vi "VisBx Anzeige.vi"() -> ()   [LabVIEW 2020, in "Anlagenuebersicht.lvlib"]
uses:
  Seiten/Anlagenuebersicht/VisBx Anzeige/Anlagenuebersicht.lvlib
  Visualisierungs Elemente/Zahlen-Ausgabefeld.ctl
  Seiten/Anlagenuebersicht/Aktionen Ausgabefaelder einfaerben.ctl
  <vilib>/Utility/miscctls.llb/LVPointTypeDef.ctl
  Seiten/Anlagengrenzwerte/FGV Anlagengrenzwerte Aktionen.ctl
  Seiten/FT-IR/FGV FT-IR Gasliste Aktionen.ctl
  PNS/Aktionen FGV Grenzwerte.ctl
  Seiten/System Einstellungen V2/Aktioen FGV System.ctl
  Seiten/FT-IR/FGV FT-IR Diagnose Aktionen.ctl
  Messdaten/Aktionen FGV Messdaten.ctl
  Amium PNS/Aktion FGV Amium Daten.ctl
  PNS/Aktionen FGV Istwerte.ctl
  Stoerungen/Stoerungen Messgeraet/Aktionen Kommunikation Stoerung.ctl
  Funktionstasten/FGV Erweiterte Bedienung Aktion.ctl
  <vilib>/picture/picture.llb/Draw True-Color Pixmap.vi
  Seiten/Erweiterte Konfig/Konfig CG-Check/CG-Test.vi
  Seiten/Anlagenuebersicht/VisBx Anzeige/VisBx Anzeige.lvlib
  Seiten/Anlagenuebersicht/VisBx Anzeige/TDMS laden/TDMS laden.lvlib
  Allgemein/allgemeine Sub-VIs.lvlib
  cRIO/PC/Kommunikation mit cRIO.lvlib
  Seiten/FT-IR/FT-IR.lvlib
  Stoerungen/Stoerungen.lvlib
  Seiten/Anlagengrenzwerte/Anlagengrenzwerte.lvlib
  Funktionstasten/Funktionstasten.lvlib
  Messdaten/Messdaten.lvlib
  PNS/PNS.lvlib
  Seiten/System Einstellungen V2/System Einstellungen V2.lvlib
  Seiten/Erweiterte Konfig/Konfig CG-Check/CG-Check Konfig.lvlib
  Amium PNS/Amium PNS.lvlib
  Amium PNS/Anlagenuebersicht_amium2.vi
panel:
  out "16B1":string="LS\n\n-16B1" caption="-21Y8"
  out "N2Exh 2":string="N2\nEXH"
  out "-22Y3 50l 2":string="-22Y3" caption="-21Y8"
  out "17B3 50l":string="LS\n\n-17B3" caption="-21Y8"
  out "17B2 50l":string="LS\n\n-17B2" caption="-21Y8"
  out "16B2 50l":string="LS\n\n-16B2" caption="-21Y8"
  out "16B2":string="LS\n\n-16B2" caption="-21Y8"
  out "-22Y1 50l":string="-22Y1" caption="-21Y8"
  out "-22Y1":string="-22Y1" caption="-21Y8"
  out "PR0,2":string="PR\n0,3bar"
  out "PA3":string="PA\n3"
  out "N2Exh":string="N2\nEXH"
  out "-23Y8":string="-23Y8"
  out "-21Y7":string="-21Y7"
  out "-21Y8":string="-21Y8"
  out "Umgebungstemperatur:":T1 format="%.1f"
  out "Boolesch":bool
  out "HL Ext. SP1:":T1 format="%.1f"
  in  "VFS":bool
  in  "VFS - Inaktiv":bool
  in  "VFS - FEHLER":bool
  in  "VFS - Aktiv":bool=TRUE
  out "kPa":T1 caption="Messgasdruck Amium"
  out "Durchflussblock":T1 caption="Durchflussblock:" format="%.1f"
  out "Druck Filterblock:":T1
  in  "CG-Test":bool caption="Dichtheitstest"
  out "Umgebungsdruck:":T1
  out "Druck Ausgang:":T1
  out "Durchfluss Bypass:":T1 caption="Flow Bypass:" format="%.1f"
  out "HL zu FID:":T1 format="%.1f"
  out "Filterblock PNS":T1 caption="Filterblock:" format="%.1f"
  out "Heizleitung SP2:":T1 caption="HL SP2:" format="%.1f"
  out "Heizleitung SP1:":T1 caption="HL SP1:" format="%.1f"
  out "Gaskühler 2":T1 caption="Gaskühler:" format="%.1f"
  out "Gaskühler":T1 caption="Gaskühler:" format="%.1f"
  out "Flow PMA:":T1 caption="Fluss PMD:" format="%.1f"
  out "Taupunkt":T1 caption="Taupunkt:" format="%.1f"
  out "Druck Kalter Block":T1 caption="Druck Kalter Block:"
  out "O2":T1 caption="O2:" format="%.2f"
  out "H2O":T1 format="%.2f"
  out "HC":T1 caption="HC:"
  in  "N2 zu PNS":bool
  out "Heizung VFE2:":T1 format="%.1f"
  out "HL Ext. SP2:":T1 format="%.1f"
  out "Schaltschrank:":T1 format="%.1f"
  out "Druck CalGas:":T1 format="%.1f"
  out "HL zu Filter:":T1 format="%.1f"
  out "HL zu FT-IR:":T1 format="%.1f"
  out "Filter:":T1 format="%.1f"
  out "Pumpe:":T1 format="%.1f"
  out "Betriebsstunden Pumpe:":T1 format="%.1f"
  out "Betriebsstunden Anlage:":T1 caption="Betriebsstunden Anlage / FTIR:" format="%.1f"
  out "Temp. Messzelle:":T1 format="%.1f"
  out "Eingangsdruck FT-IR:":T1 format="%.3f"
  out "Durchfluss FT-IR:":T1 format="%.1f"
  out "Aktive Störungen":string[](array[string])
  in  "Fehler":string="Die Umgebungsvariable besitzt\nnicht den selben Datentyp wie\ndie TDMS-Datei."
  out "Bild":picture
  # "Anlagenübersicht"
  # "SPAN 1"
  # "-23Y1"
  # "SPAN 2"
  # "-23Y6"
  # "PS"
  # "-23Y2"
  # "SPAN 3"
  # "0-10"
  # "bar"
  # "-22Y2"
  # "-23Y3"
  # "-35B5"
  # "N2.....Stickstoff Gasförmig\nCA.....Druckluft\nCG.....Cal. Gas\nAA.....Umgebungs Luft\nPA.....Spülluft FT-IR\n\nPR....Druckregler\nPS....Druckschalter\nFS....Flow Regler\nLS....Levelsensor\nFM...Flow Sensor"
  # "-35B1"
  # "-23Y4"
  # "FM"
  # "-43Y1"
  # "S"
  # "-21Y5"
  # "FTIR"
  # "-35B2"
  # "-11Y7"
  # "-11Y3"
  # "SP1"
  # "-11Y5"
  # "-11Y6"
  # "SP2"
  # "-11Y2"
  # "-12Y1"
  # "-11Y8"
  # "Absaugung"
  # "7A1"
  # "P out"
  # "CA to PNS"
  # "-17B8"
  # "Druckluft"
  # "min 4bar"
  # "-20Y1"
  # "PR01"
  # "-17S1"
  # "Purge in"
  # "Druckspeicher 5l"
  # "-20Y8"
  # "°C"
  # "°C"
  # "-44Y1"
  # "-21Y8"
  # "-23Y8"
  # "-21Y7"
  # "°C"
  # "mbar"
  # "-10M2"
  # "-20Y2"
  # "°C"
  # "-20Y4"
  # "-20Y6"
  # "-7M8"
  # "-35B10"
  # "-35B6"
  # "N2"
  # "1-2"
  # "LS"
  # "°C"
  # "CA"
  # "6"
  # "N2"
  # "1-2"
  # "N2"
  # "3"
  # "CA"
  # "1-2"
  # "EPR"
  # "5bar"
  # "CA"
  # "1"
  # "N2"
  # "2"
  # "CA"
  # "2"
  # "N2"
  # "4"
  # "CA"
  # "PNS"
  # "CG"
  # "PNS"
  # "N2"
  # "3-4"
  # "CG"
  # "PNS"
  # "FID"
  # "EXH"
  # "°C"
  # "°C"
  # "mbar"
  # "mbar"
  # "l/min"
  # "°C"
  # "FID"
  # "EXH"
  # "M2"
  # "PR02"
  # "PR"
  # "4bar"
  # "CA"
  # "FID"
  # "M6"
  # "PR06"
  # "M7"
  # "PR07"
  # "H2"
  # "FID"
  # "PR"
  # "1,2bar"
  # "SA"
  # "FID"
  # "PR"
  # "1,2bar"
  # "-27Y4"
  # "-27Y3"
  # "PR09"
  # "-35B8"
  # "CG"
  # "O2"
  # "PS"
  # "3,5bar"
  # "FR"
  # "1,5l"
  # "FID"
  # "FID"
  # "EXH"
  # "4 bar"
  # "CA"
  # "1,2bar"
  # "H2"
  # "1,2bar"
  # "SA"
  # "SPAN 2"
  # "SPAN 3"
  # "°C"
  # "°C"
  # "°C"
  # "°C"
  # "°C"
  # "l/min"
  # "°C"
  # "mbar"
  # "H"
  # "S"
  # "P"
  # "abs"
  # "PMA"
  # "%"
  # "-35B9"
  # "FM"
  # "S"
  # "-27Y2"
  # "CG O2"
  # "CG"
  # "O2"
  # "%"
  # "ppm"
  # "°C"
  # "°C"
  # "°C"
  # "bar"
  # "°C"
  # "°C"
  # "°C"
  # "°C"
  # "h"
  # "h"
  # "°C"
  # "atm"
  # "l/min"
  # "N2"
  # "1"
  # "PR"
  # "2bar"
  # "PS"
  # "1bar"
  # "PR"
  # "5bar"
  # "PS"
  # "4bar"
  # "FS"
  # "3l"
  # "PR51"
  # "P"
  # "abs"
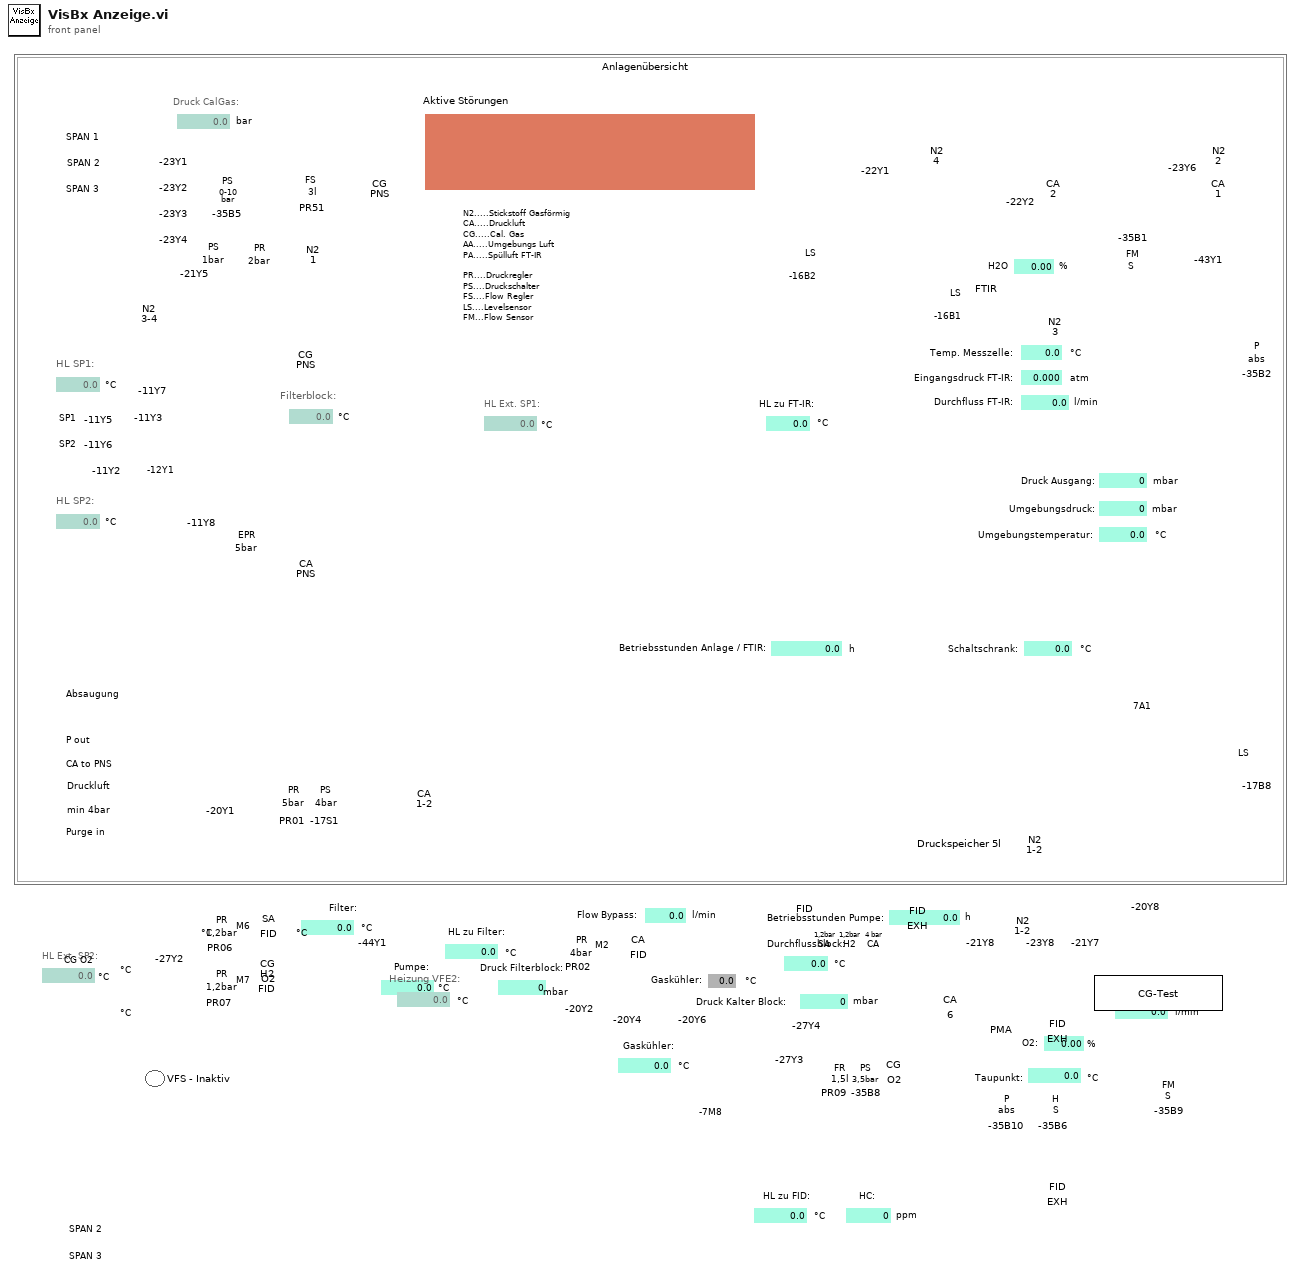
[diagram p1: front panel]
types:
  T1 = typedef "Zahlen-Ausgabefeld.ctl" = sgl
  T2 = typedef "System Einstellungen V2.lvlib/Aktioen FGV System.ctl" = enum16{"lesen", "laden", "speichern", "Optionen schreiben", "Zeitstempel", "Reset BMP", "Reset SQP", "Wartung", "Werkseinstellung"}
  T3 = typedef "PNS.lvlib/Aktionen FGV Grenzwerte.ctl" = enum16{"lesen", "Grenzw. schreiben", "Anweisungscode", "IP-Adresse", "laden", "speichern", "Anweisungscode vorgeben"}
  T4 = typedef "FT-IR.lvlib/FGV FT-IR Gasliste Aktionen.ctl" = enum16{"lesen", "Gasliste FT-IR", "Gasliste ausgelesen", "laden", "speichern", "löschen"}
  T5 = typedef "Anlagengrenzwerte.lvlib/FGV Anlagengrenzwerte Aktionen.ctl" = enum16{"Lesen", "Grenzwerte schreiben"}
  T6 = typedef "LVPointTypeDef.ctl" = cluster{"Horizontal":i16, "Vertical":i16}
  T7 = typedef "Anlagenuebersicht.lvlib/Aktionen Ausgabefaelder einfaerben.ctl" = enum16{"lesen", "prüfen", "initialisieren"}
  T8 = typedef "Funktionstasten.lvlib/FGV Erweiterte Bedienung Aktion.ctl" = enum16{"Lesen", "Initialisieren", "N2 zu PNS", "Chart wechsel"}
  T9 = enum8{"Enabled", "Disabled", "Disabled and Grayed Out"}
  T10 = typedef "Steuerung PNS.lvclass/Anlegengrenzwerte PNS.ctl" = cluster{"Filter:":T11, "Ventilplatte:":T11, "Heizleitung 1:":T11, "Heizleitung 2:":T11, "Heizleitung 3:":T11, "Heizleitung 4:":T11, "Heizleitung 5:":T11, "Heizleitung 6:":T11}
  T11 = typedef "Steuerung PNS.lvclass/Anlagengrenzwerte Parameteranzeige.ctl" = cluster{"Sollwert":T12, "Warn-Min":T12, "Warn-Max":T12, "Abschalt-Min":T12, "Abschalt-Max":T12, "Regler":u16, "AnlagenParameter":string}
  T12 = typedef "Zahlen-Eingabefeld.ctl" = sgl
  T13 = typedef "Anlagengrenzwerte.lvlib/Anlagen-Grenzwerte Anzeige.ctl" = cluster{"Eingangsdruck FT-IR:":T14, "Durchfluss FT-IR:":T14, "Durchfluss CalGas:":T14, "Druck Ausgang:":T14, "Druck Kalter Block:":T14, "Heizleitungen intern:":T14, "Heizleitung zu FT-IR:":T14, "Heizung Filterblock:":T14, "Heizung Pumpe:":T14, "Heizleitung Extern SP1:":T14, "Heizleitung Extern SP2:":T14, "FT-IR Heizung Messzelle:":T14, "Schaltschranktemperatur:":T14, "Gaskühler:":T14}
  T14 = typedef "Anlagengrenzwerte.lvlib/Anlagen-Parameter Anzeige.ctl" = cluster{"Sollwert":sgl, "Warn-Min":sgl, "Warn-Max":sgl, "Abschalt-Min":sgl, "Abschalt-Max":sgl, "Regler":u16}
  T15 = typedef "System Einstellungen V2.lvlib/Optionen.ctl" = cluster{"Störmeldep.":bool, "Betriebszustände":bool, "AK in ppm":bool, "log Cal-Gas":bool, "log 0-Gas":bool, "Durchflusssensor 0-5V":bool, "PNS?":bool, "Mit N2 spülen":bool, "TRE08":bool, "Amium 10-Fach":bool, "Verticale Scrollbar aktiv":bool, "Loggingtakt":bool, "AK Rezeptwechsel gleich wie MKS":bool, "NG ECO":bool}
  T16 = typedef "VisParam-Typdef.lvlib/VisSchritt.ctl" = cluster{"Schritt-Typ":T17, "Schritt-Daten":variant}
  T17 = typedef "VisParam-Typdef.lvlib/VisSchritt-Typ.ctl" = enum16{"leer", "Punkt", "Linie", "Linienzug", "Fixtext", "Textrechteck", "Ziffernanzeige", "Rechteck", "Rechteck rund", "Ellipse", "Bogen", "Kreis", "Pixmap"}
  T18 = typedef "Anlagenuebersicht.lvlib/VisBx Anzeige.lvlib/TDMS laden.lvlib/TDMS-Eigenschaften.ctl" = cluster{"Größe":T19, "URL":string, "Raster":i16, "Hintergrund":u32}
  T19 = typedef "LVBoundsTypeDef.ctl" = cluster{"Width":u32, "Height":u32}
  T20 = typedef "String - Ausgabefeld.ctl" = string
  T21 = typedef "PNS.lvlib/Aktionen FGV Istwerte.ctl" = enum16{"lesen", "initialisieren", "schreiben", "Störungen"}
  T22 = typedef "Amium PNS.lvlib/Aktion FGV Amium Daten.ctl" = enum16{"lesen", "Komm Daten", "Daten", "Error", "Regler", "Grenzwerte", "laden", "speichern"}
  T23 = typedef "Messdaten.lvlib/Aktionen FGV Messdaten.ctl" = enum16{"lesen", "schreiben", "löschen", "Mittelwerte", "Komponente"}
  T24 = typedef "FT-IR.lvlib/FGV FT-IR Diagnose Aktionen.ctl" = enum16{"Lesen", "Diagnose Schreiben", "Min Schreiben", "Max Schreiben"}
  T25 = typedef "Stoerungen.lvlib/Aktionen Kommunikation Stoerung.ctl" = enum16{"lesen", "init", "FT-IR Komm", "FT-IR Betriebsart", "FT-IR Hintergrund", "cRIO Komm", "PNS Komm", "Dichtheitstest", "Life Bit", "FTIR Komm AK", "PMA Komm", "FID Komm", "PMA Cal", "FID Ch4 Cal", "FID THC Cal", "Cal Timeout", "VFS 1 Komm", "VFS 2 Komm", "VFS 3 Komm", "VFS 4 Komm", "TRE 08 Komm", "CG-Test vorzeitig", "CG-Test Span 1", "CG-Test Span 2", "CG-Test Span 3", "CG-Test Messgas", "CG-Test löschen", "Test", "Amium AK", "AK Recept konfig", "AK Name konfig", "AK EKFG konfig"}
  T26 = typedef "Stoerungen.lvlib/Stoerungen Messgeraete.ctl" = cluster{"FT-IR Komm":bool, "FT-IR Betriebsart":bool, "FT-IR Hintergrundscan":bool, "Dichtheitstest":bool, "cRIO Komm":bool, "PNS Komm":bool, "Life Bit":bool, "FT-IR AK Komm":bool, "PMA Komm":bool, "FID Komm":bool, "PMA Cal":bool, "FID CH4 Cal":bool, "FID THC Cal":bool, "Cal Timeout":bool, "VFS 1 Komm":bool, "VFS 2 Komm":bool, "VFS 3 Komm":bool, "VFS 4 Komm":bool, "TRE 08 Komm":bool, "CG-Test":bool, "CG-Test 1":bool, "CG-Test 2":bool, "CG-Test 3":bool, "Messgas - Eingang":bool, "Amium AK Komm":bool, "AK Rezept nicht konfiguriert ":bool, "AK Name nicht konfiguriert":bool, "AK EKFG nicht konfiguriert":bool}
  T27 = typedef "Steuerung PNS.lvclass/Regler.ctl" = cluster{"Istwert":i16, "Sollwert":i16, "Alarm MIN":i16, "Alarm MAX":i16, "Regler sperren":i16, "Analog Ausgang":i16}[]
  T28 = typedef "Verwaltung - cRIO.lvlib/Analog Eingaenge.ctl" = cluster{"AI0: Durchfluss FT-IR":sgl, "AI1: Druck Ausgang":sgl, "AI2: Umgebungsdruck":sgl, "AI3: Druck FT-IR":sgl, "AI4: Druck CalGas":sgl, "AI5: Reserve":sgl, "AI6: Reserve":sgl, "AI7: Reserve":sgl, "Rohwert Durchfluss FT-IR":sgl, "Rohwert Druck Ausgang":sgl, "Rohwert Umgebungsdruck":sgl, "Rohwert Druck FT-IR":sgl, "Rohwert Druck CalGas":sgl, "Rohwert AI5":sgl, "Rohwert AI6":sgl, "Rohwert AI7":sgl, "Rohwert Diffdruck mbar FTIR":sgl}
  T29 = typedef "Verwaltung - cRIO.lvlib/TC Eingaenge.ctl" = cluster{"TC0: Reserve":sgl, "TC1: HL zu FT-IR":sgl, "TC2: HL Extern SP1":sgl, "TC3: HL Extern SP2":sgl, "TC4: Reserve":sgl, "TC5: Reserve":sgl, "TC6: Reserve":sgl, "TC7: Reserve":sgl, "TC8: FT-IR":sgl, "TC9: Reserve":sgl, "TC10: Schaltschrank":sgl, "TC11: Umgebung":sgl}
  T30 = typedef "Amium PNS.lvlib/Daten Cluster.ctl" = cluster{"Amium Zustände":T31, "Samplepoint am PNS":i16, "Gerätekennung":string, "aktiver Samplepoint":i16[], "Messgasdruck":sgl}
  T31 = typedef "Amium PNS.lvlib/Amium Zustand.ctl" = u16
  T32 = cluster{"Istwert":i16, "Sollwert":i16, "Alarm MIN":i16, "Alarm MAX":i16, "Regler sperren":i16, "Analog Ausgang":i16}
  T33 = typedef "Verwaltung - cRIO.lvlib/Digital Ausgaenge 0-31.ctl" = cluster{"O0: Druckluft Versorgung":bool, "O1: CG 1 (FB Eingang 1)":bool, "O2: CG 2 (Kühlung FT-IR EIN)":bool, "O3: CG 3 (FB Bypass)":bool, "O4: CG 4 (FB CalGas)":bool, "O5: CG 5 (FB spülen/UL)":bool, "O6: CG 6 (FB zum FT-IR)":bool, "O7: CG 7 (FB zum FID)":bool, "O8: CG 8 (FB Reserve)":bool, "O9: (FB Reserve)":bool, "O10: (FB Umgebungsluft FID)":bool, "O11: (FB zum Gaskühler)":bool, "O12: FB Stickstoff zu FT-IR":bool, "O13: Optikbox FT-IR spülen":bool, "O14: (Purifier deaktivieren)":bool, "O15: (Umschaltung Purifier/Stickstoff)":bool, "O16: N2 Einblasung":bool, "O17: LSP LN2 Nachfüllung":bool, "O18: (Reserve)":bool, "O19: (Pumpe Eingang1)":bool, "O20: (Pumpe Eingang2)":bool, "O21: (Pumpe Spülen1)":bool, "O22: (Pumpe Spülen2)":bool, "O23: (Reserve)":bool, "O24: CalGas 1":bool, "O25: CalGas 2":bool, "O26: CG 3-8 (CalGas 3)":bool, "O27: Stickstoff aufschalten":bool, "O28: CG zu PNS":bool, "O29: FTIR Standby Spülung":bool, "O30: CG zu Entnahme(T90)":bool, "O31: (Purifier regenerieren)":bool}
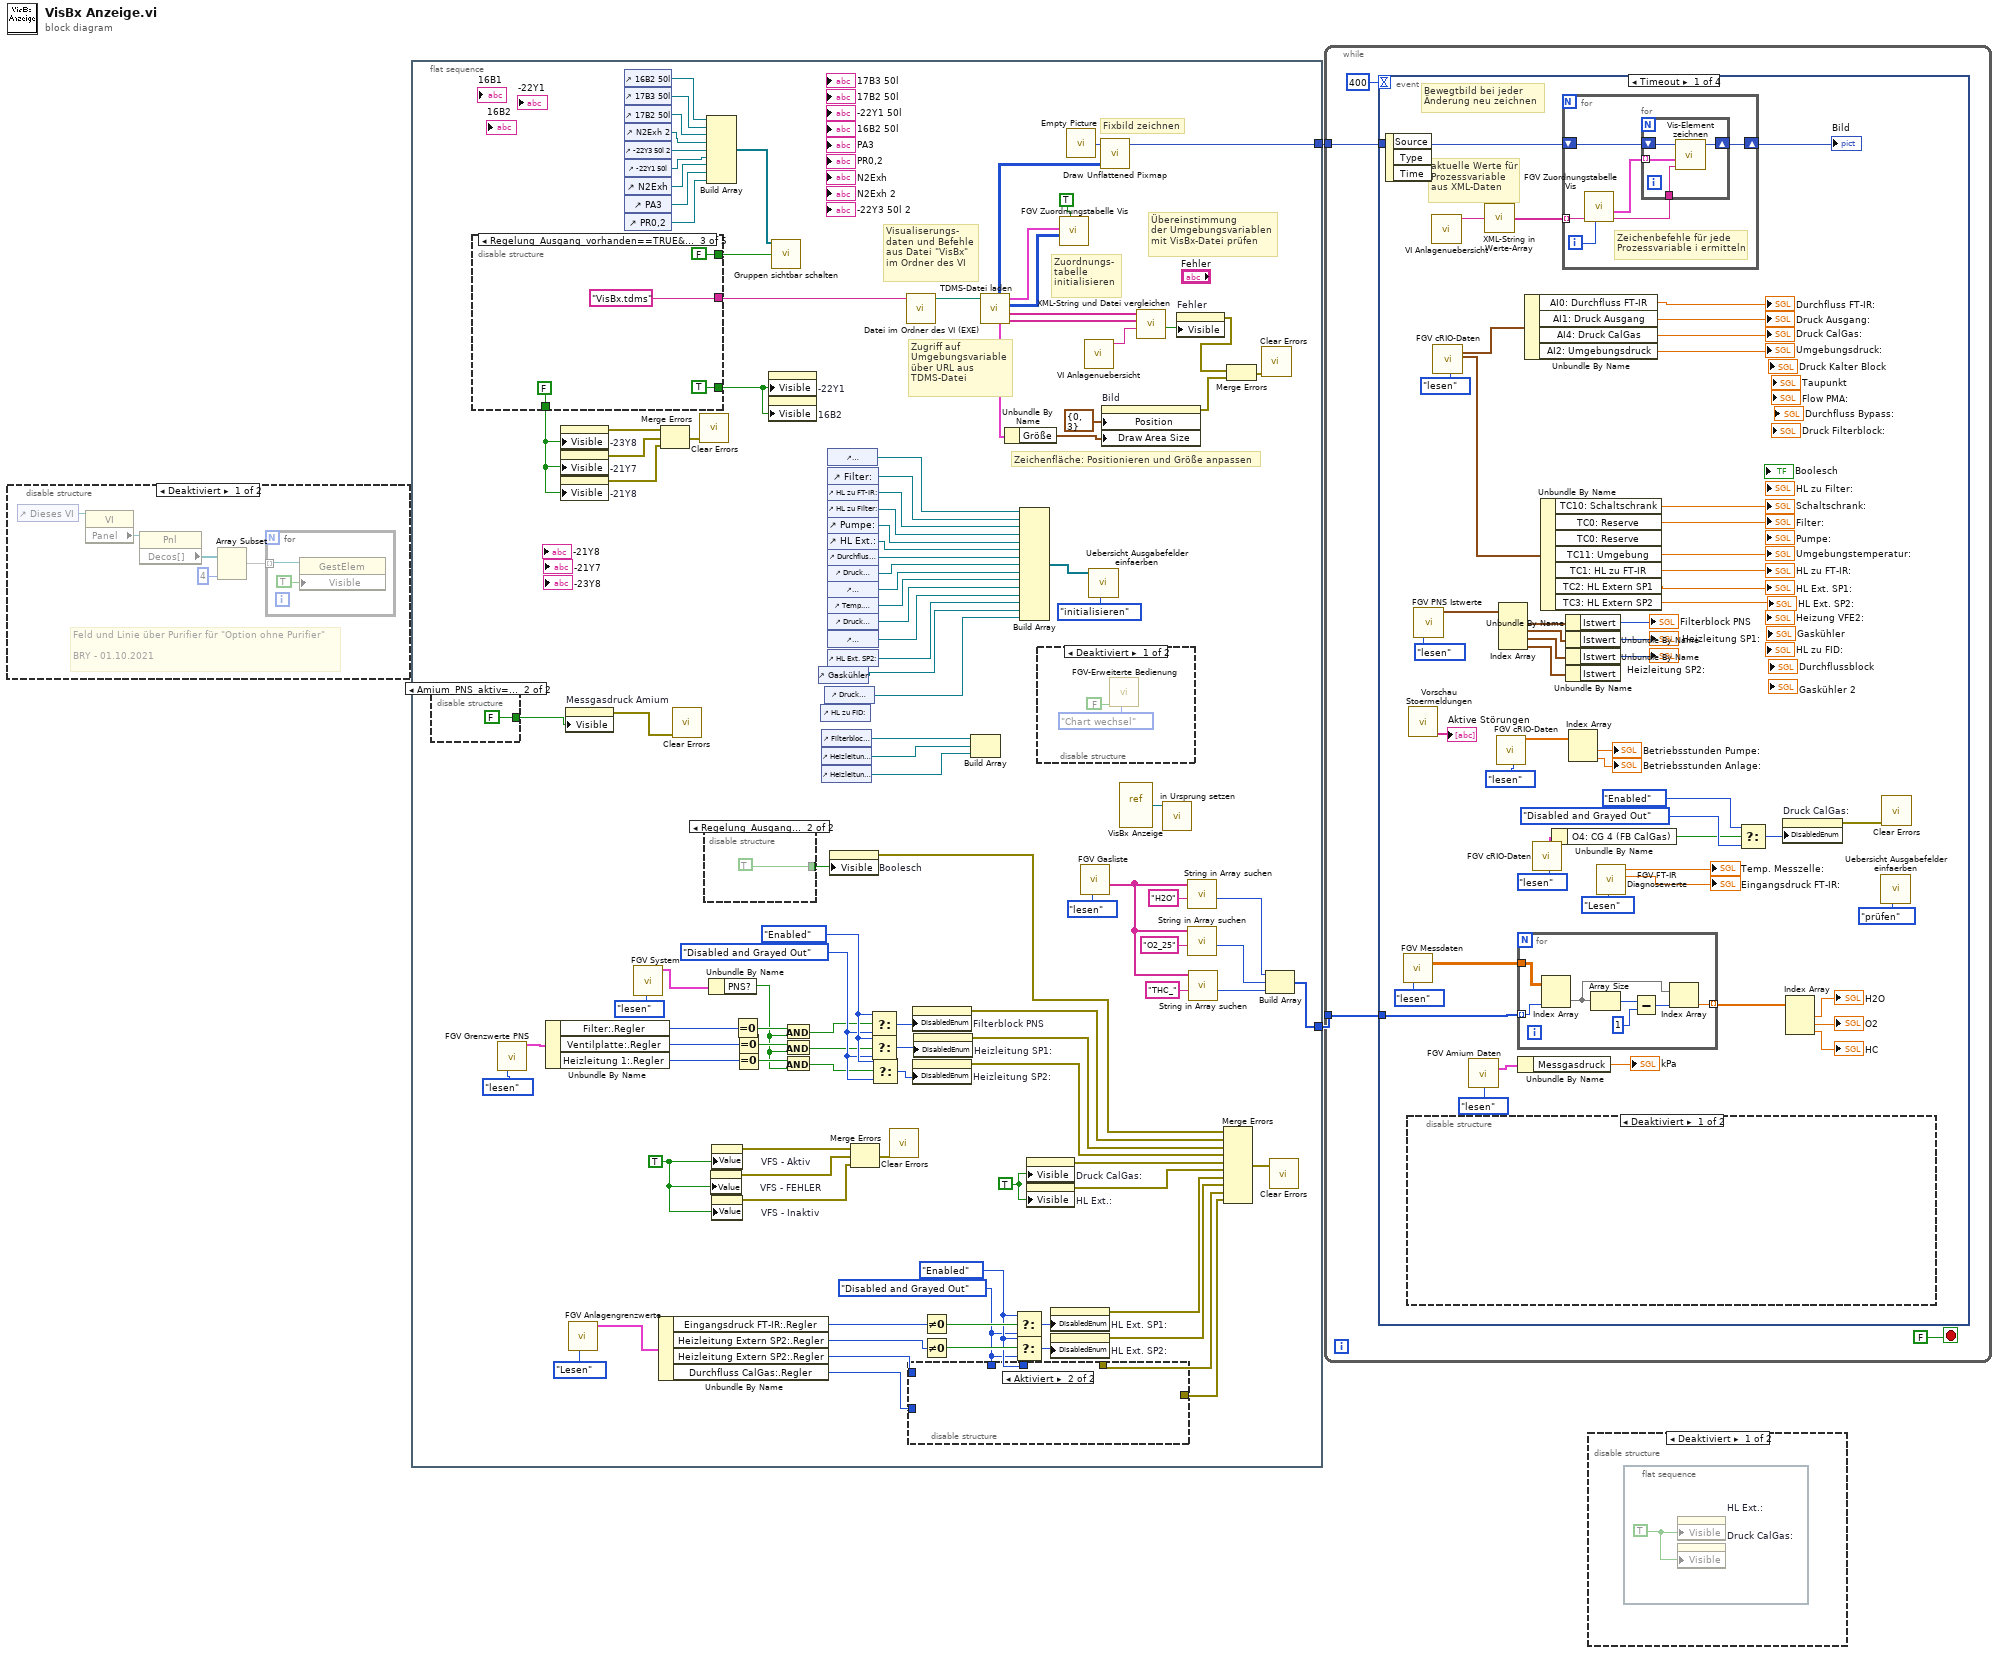
[diagram p0: block diagram]
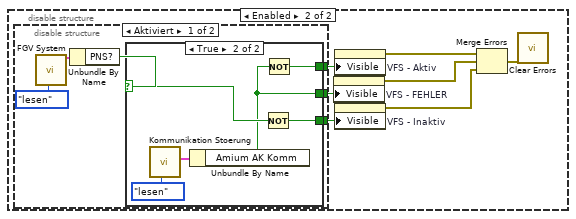
[diagram p4: hidden frame]
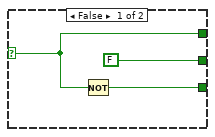
[diagram p5: hidden frame]
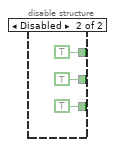
[diagram p6: hidden frame]
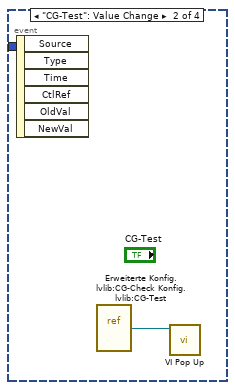
[diagram p7: hidden frame]
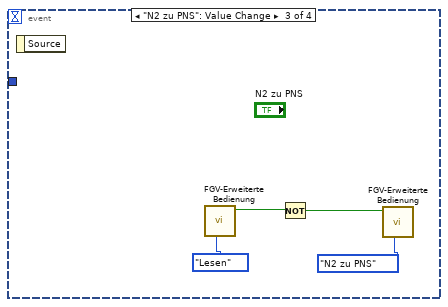
[diagram p8: hidden frame]
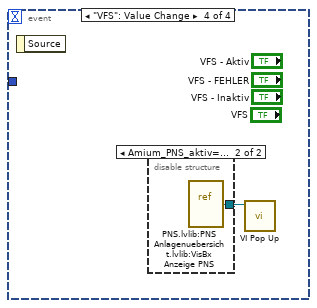
[diagram p9: hidden frame]
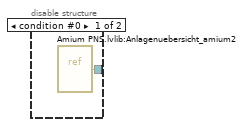
[diagram p10: hidden frame]
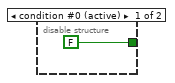
[diagram p11: hidden frame]
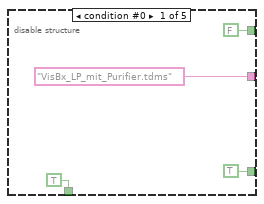
[diagram p12: hidden frame]
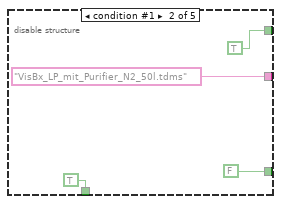
[diagram p13: hidden frame]
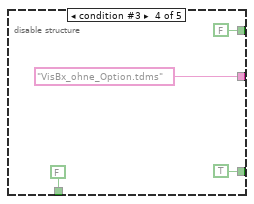
[diagram p14: hidden frame]
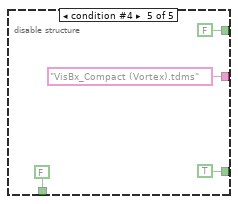
[diagram p15: hidden frame]
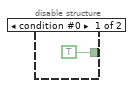
[diagram p16: hidden frame]
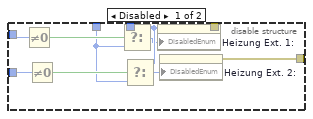
[diagram p17: hidden frame]
diagram:
  n1 = disable-structure shown="Deaktiviert" {
    frame Disabled {
      # "Feld und Linie über Purifier für \"Option ohne Purifier\"\n\nBRY - 01.10.2021"
      n2 = control-ref of="Dieses VI"() -> (w7:refnum<vi>)
      n3 = property class="VI"(reference=w7) -> ("Panel"=w6:refnum<vi>)  [unwired: 1 in, 2 out]
      n4 = property class="Pnl"(reference=w6) -> ("Decos[]"=w5:refnum<vi>[])  [unwired: 1 in, 2 out]
      n5 = Array Subset(array=w5, length=4 ("Länge")) -> (w3:refnum<vi>[])  [unwired: 1 in]
      n6 = for {
        tunnel: w3 -> [w9] mode=indexing
        n7 = property class="GestElem"(reference=w9, "Visible"=TRUE ("Sichtbar")) -> ()  [unwired: 1 in, 2 out]
      }
    }
    frame Enabled {
    }
  }
  n8 = flat-sequence {
    tunnel: [w99] -> w2
    tunnel: [w66] -> w1
    frame #0 {
      w32 = TRUE ("Sichtbar")
      w51 = T9."Enabled" ("t")
      w50 = T9."Disabled and Grayed Out" ("Deaktiviert")
      w80 = T9."Enabled" ("t")
      w79 = T9."Disabled and Grayed Out" ("Deaktiviert")
      w92 = TRUE ("Sichtbar")
      # "Übereinstimmung\nder Umgebungsvariablen\nmit VisBx-Datei prüfen"
      # "Zugriff auf\nUmgebungsvariable\nüber URL aus\nTDMS-Datei"
      # "Visualiserungs-\ndaten und Befehle\naus Datei \"VisBx\"\nim Ordner des VI"
      # "Zuordnungs-\ntabelle\ninitialisieren"
      # "Zeichenfläche: Positionieren und Größe anpassen"
      # "Fixbild zeichnen"
      n9 = disable-structure shown="Amium_PNS_aktiv==FALSE, Standard" {
        disable-tunnel: [TRUE FALSE] -> w31
        frame condition #0 {
        }
        frame condition #1 (active) {
        }
      }
      n10 = disable-structure shown="Regelung_Ausgang_vorhanden==TRUE&&LN2_Befuellung==TRUE&&Purifier==FALSE&&50l_N2_Tank==FALSE" {
        disable-tunnel: ["VisBx_LP_mit_Purifier.tdms" ("Dateiname") "VisBx_LP_mit_Purifier_N2_50l.tdms" ("Dateiname") "VisBx.tdms" ("Dateiname") "VisBx_ohne_Option.tdms" ("Dateiname") "VisBx_Compact (Vortex).tdms" ("Dateiname")] -> w29
        disable-tunnel: [TRUE ("Sichtbar") TRUE ("Sichtbar") FALSE ("Sichtbar") FALSE ("Sichtbar") FALSE ("Sichtbar")] -> w26
        disable-tunnel: [TRUE ("Sichtbar") FALSE ("Sichtbar") TRUE ("Sichtbar") TRUE ("Sichtbar") TRUE ("Sichtbar")] -> w21
        disable-tunnel: [FALSE ("Sichtbar") TRUE ("Sichtbar") FALSE ("Sichtbar") FALSE ("Sichtbar") FALSE ("Sichtbar")] -> w10
        frame condition #0 {
        }
        frame condition #1 {
        }
        frame condition #2 (active) {
        }
        frame condition #3 {
        }
        frame condition #4 {
        }
      }
      n11 = call "FGV Grenzwerte PNS.vi"("Aktionen FGV Grenzwerte"=Aktionen_FGV_Grenzwerte."lesen") -> ("Grenzwerte PNS 2"=w62:T10)  [unwired: 12 in, 2 out]
      n12 = Unbundle By Name(w62) -> ("Filter:.Regler"=w60:u16, "Ventilplatte:.Regler"=w59:u16, "Heizleitung 1:.Regler"=w58:u16)
      n13 = property on="-23Y8" class="Str"("Visible"=w26) -> (error out=w25:errorcluster)  [unwired: 2 in, 1 out]
      n14 = property on="-21Y7" class="Str"("Visible"=w26) -> (error out=w24:errorcluster)  [unwired: 2 in, 1 out]
      n15 = property on="-21Y8" class="Str"("Visible"=w26) -> (error out=w23:errorcluster)  [unwired: 2 in, 1 out]
      n16 = property on="Messgasdruck Amium" class="DigWert (strikt)"("Visible"=w31) -> (error out=w30:errorcluster)  [unwired: 2 in, 1 out]
      n17 = call "FGV Anlagengrenzwerte.vi"("Aktion"=FGV_Anlagengrenzwerte_Aktionen."Lesen") -> ("Anlagen-Grenzwerte Anzeige"=w89:T13)  [unwired: 1 in, 9 out]
      n18 = control-ref of="16B2 50l"() -> (w20:refnum<vi>)
      n19 = control-ref of="17B3 50l"() -> (w19:refnum<vi>)
      n20 = control-ref of="17B2 50l"() -> (w18:refnum<vi>)
      n21 = control-ref of="N2Exh 2"() -> (w17:refnum<vi>)
      n22 = control-ref of="-22Y3 50l 2"() -> (w16:refnum<vi>)
      n23 = control-ref of="-22Y1 50l"() -> (w15:refnum<vi>)
      n24 = control-ref of="N2Exh"() -> (w14:refnum<vi>)
      n25 = control-ref of="PA3"() -> (w13:refnum<vi>)
      n26 = control-ref of="PR0,2"() -> (w12:refnum<vi>)
      n27 = call "FGV System.vi"("Aktionen"=Aktioen_FGV_System."lesen") -> ("Optionen"=w53:T15)  [unwired: 12 in, 6 out]
      n28 = Unbundle By Name(w89) -> ("Eingangsdruck FT-IR:.Regler"=w87:u16, "Heizleitung Extern SP2:.Regler"=w83:u16, "Heizleitung Extern SP2:.Regler"=w81:u16, "Durchfluss CalGas:.Regler"=w78:u16)
      n29 = Merge Errors(w25, w24, w23) -> (w22:errorcluster)
      n30 = call <vilib>:"Clear Errors.vi"("error in (no error)"=w30) -> ()  [unwired: 5 in, 2 out]
      n31 = call <vilib>:"Clear Errors.vi"("error in (no error)"=w22) -> ()  [unwired: 5 in, 2 out]
      n32 = disable-structure shown="Regelung_Ausgang_vorhanden==FALSE" {
        disable-tunnel: [FALSE ("Sichtbar") TRUE ("Sichtbar")] -> w28
        frame condition #0 (active) {
        }
        frame condition #1 {
        }
      }
      n33 = Build Array(w20, w19, w18, w17, w16, w15, w14, w13, w12) -> (w11:refnum<vi>[])
      n34 = Unbundle By Name(w53) -> ("PNS?"=w52:bool)
      n35 = property on="VFS - FEHLER" class="Bool. (strikt)"("Value"=w32) -> (error out=w34:errorcluster)  [unwired: 2 in, 1 out]
      n36 = property on="VFS - Aktiv" class="Bool. (strikt)"("Value"=w32) -> (error out=w35:errorcluster)  [unwired: 2 in, 1 out]
      n37 = property on="VFS - Inaktiv" class="Bool. (strikt)"("Value"=w32) -> (error out=w33:errorcluster)  [unwired: 2 in, 1 out]
      n38 = Equal To 0?(x=w60) -> (x = 0?=w57:bool)
      n39 = Equal To 0?(x=w59) -> (x = 0?=w56:bool)
      n40 = Equal To 0?(x=w58) -> (x = 0?=w55:bool)
      n41 = property on="-22Y1" class="Str"("Visible"=w21) -> ()  [unwired: 2 in, 2 out]
      n42 = property on="16B2" class="Str"("Visible"=w21) -> ()  [unwired: 2 in, 2 out]
      n43 = call "Gruppen sichtbar schalten.vi"("Element Referenzen"=w11, "Sichtbar"=w10) -> ()  [unwired: 13 in, 1 out]
      n44 = And(x=w57, y=w52) -> (x .and. y?=w49:bool)
      n45 = And(x=w56, y=w52) -> (x .and. y?=w48:bool)
      n46 = And(x=w55, y=w52) -> (x .and. y?=w47:bool)
      n47 = control-ref of="Gaskühler"() -> (w63:refnum<vi>)
      n48 = control-ref of="HL zu FID:"() -> ()  [unwired: 1 out]
      n49 = control-ref of="Filterblock PNS"() -> (w40:refnum<vi>)
      n50 = control-ref of="Heizleitung SP1:"() -> (w39:refnum<vi>)
      n51 = control-ref of="Heizleitung SP2:"() -> (w38:refnum<vi>)
      n52 = control-ref of="Druck Kalter Block"() -> (w64:refnum<vi>)
      n53 = control-ref of="Durchflussblock"() -> (w37:refnum<vi>)
      n54 = control-ref of="Filter:"() -> (w123:refnum<vi>)
      n55 = control-ref of="HL zu FT-IR:"() -> (w125:refnum<vi>)
      n56 = control-ref of="HL zu Filter:"() -> (w124:refnum<vi>)
      n57 = control-ref of="Pumpe:"() -> (w122:refnum<vi>)
      n58 = control-ref of="HL Ext.:"() -> (w121:refnum<vi>)
      n59 = control-ref of="Durchfluss FT-IR:"() -> (w120:refnum<vi>)
      n60 = control-ref of="Druck Ausgang:"() -> (w119:refnum<vi>)
      n61 = control-ref of="Eingangsdruck FT-IR:"() -> (w118:refnum<vi>)
      n62 = control-ref of="Temp. Messzelle:"() -> (w117:refnum<vi>)
      n63 = control-ref of="Druck CalGas:"() -> (w114:refnum<vi>)
      n64 = control-ref of="Schaltschrank:"() -> (w91:refnum<vi>)
      n65 = control-ref of="HL Ext. SP2:"() -> (w74:refnum<vi>)
      n66 = property on="Boolesch" class="Bool. (strikt)"("Visible"=w28) -> (error out=w27:errorcluster)  [unwired: 2 in, 1 out]
      n67 = Merge Errors(w35, w34, w33) -> (w36:errorcluster)
      n68 = Select(t=w51, s=w49, f=w50) -> (s? t:f=w46:T9)
      n69 = Select(t=w51, s=w48, f=w50) -> (s? t:f=w45:T9)
      n70 = Select(t=w51, s=w47, f=w50) -> (s? t:f=w44:T9)
      n71 = call <vilib>:"Clear Errors.vi"("error in (no error)"=w36) -> ()  [unwired: 5 in, 2 out]
      n72 = call "Datei im Ordner des VI (EXE).vi"("Dateiname"=w29) -> ("Dateipfad im Ordner des Haupt-VIs"=w112:path)  [unwired: 8 in, 2 out]
      n73 = disable-structure shown="Aktiviert" {
        disable-tunnel: w81 -> [w158 _]
        disable-tunnel: w80 -> [w156 _]
        disable-tunnel: w79 -> [w155 _]
        disable-tunnel: w78 -> [w154 _]
        disable-tunnel: [w151 _] -> w76
        disable-tunnel: [w150 _] -> w75
        frame Disabled {
          n74 = Not Equal To 0?(x=w158) -> (x != 0?=w159:bool)
          n75 = Not Equal To 0?(x=w154) -> (x != 0?=w157:bool)
          n76 = Select(t=w156, s=w159, f=w155) -> (s? t:f=w153:T9)
          n77 = Select(t=w156, s=w157, f=w155) -> (s? t:f=w152:T9)
          n78 = property on="Heizung Ext. 1:" class="DigWert (strikt)"("DisabledEnum"=w153) -> (error out=w151:errorcluster)  [unwired: 2 in, 1 out]
          n79 = property on="Heizung Ext. 2:" class="DigWert (strikt)"("DisabledEnum"=w152) -> (error out=w150:errorcluster)  [unwired: 2 in, 1 out]
        }
        frame Enabled {
        }
      }
      n80 = property on="Filterblock PNS" class="DigWert (strikt)"("DisabledEnum"=w46) -> (error out=w43:errorcluster)  [unwired: 2 in, 1 out]
      n81 = property on="Heizleitung SP2:" class="DigWert (strikt)"("DisabledEnum"=w44) -> (error out=w41:errorcluster)  [unwired: 2 in, 1 out]
      n82 = property on="Heizleitung SP1:" class="DigWert (strikt)"("DisabledEnum"=w45) -> (error out=w42:errorcluster)  [unwired: 2 in, 1 out]
      n83 = Not Equal To 0?(x=w87) -> (x != 0?=w88:bool)
      n84 = Not Equal To 0?(x=w83) -> (x != 0?=w84:bool)
      n85 = Build Array(w40, w39, w38) -> ()  [unwired: 1 out]
      n86 = call "TDMS-Datei laden.vi"("Dateipfad"=w112) -> ("Datentypen"=w108:string[], "Namen"=w104:string[], "Zuordnungstabelle"=w102:i16[][], "Programm"=w103:T16[], "Eigenschaften"=w105:T18, "Fixbild (Pixmap)"=w106:u32[][])  [unwired: 5 out]
      n87 = Unbundle By Name(w105) -> ("Größe"=w111:T19)
      n88 = Select(t=w80, s=w88, f=w79) -> (s? t:f=w86:T9)
      n89 = Select(t=w80, s=w84, f=w79) -> (s? t:f=w82:T9)
      n90 = Build Array(w37, w123, w125, w124, w122, w121, w120, w119, w118, w117, w114, w91, w74, w63, w64) -> (w116:refnum<vi>[])
      n91 = property on="Druck CalGas:" class="DigWert (strikt)"("Visible"=w92) -> (error out=w93:errorcluster)  [unwired: 2 in, 1 out]
      n92 = property on="HL Ext.:" class="DigWert (strikt)"("Visible"=w92) -> (error out=w94:errorcluster)  [unwired: 2 in, 1 out]
      n93 = disable-structure shown="Deaktiviert" {
        frame Disabled {
          n94 = call "FGV-Erweiterte Bedienung.vi"("Aktion"=FGV_Erweiterte_Bedienung_Aktion."Chart wechsel", "Chart wechsel"=FALSE) -> ()  [unwired: 8 in, 2 out]
        }
        frame Enabled {
        }
      }
      n95 = property on="HL Ext. SP1:" class="DigWert (strikt)"("DisabledEnum"=w86) -> (error out=w85:errorcluster)  [unwired: 2 in, 1 out]
      n96 = property on="HL Ext. SP2:" class="DigWert (strikt)"("DisabledEnum"=w82) -> (error out=w77:errorcluster)  [unwired: 2 in, 1 out]
      n97 = call "FGV Zuordnungstabelle Vis.vi"("Initialisieren"=TRUE, "Zuordnungtabelle (init)"=w102, "Programm (init)"=w103) -> ()  [unwired: 3 in, 6 out]
      n98 = call "Empty Picture"() -> ("empty picture"=w107:picture)
      n99 = call "FGV Gasliste.vi"("Aktionen"=FGV_FT-IR_Gasliste_Aktionen."lesen") -> ("Aktuelle Gasliste gesamt"=w65:T20[])  [unwired: 8 in, 2 out]
      n100 = call "VI Anlagenuebersicht.vi"() -> ("XML-String"=w109:string)  [unwired: 11 in]
      n101 = call "Uebersicht Ausgabefelder einfaerben.vi"("Aktionen"=Aktionen_Ausgabefaelder_einfaerben."initialisieren", "Angehängtes Array"=w116) -> ()  [unwired: 10 in]
      n102 = call-poly <vilib>:"Draw Unflattened Pixmap.vi"("picture"=w107, "data (RGB format)"=w106) -> ("new picture"=w99:picture)  [unwired: 7 in]
      n103 = property on="Bild" class="Bild"("Position"=T6 {"Horizontal"=0, "Vertical"=3} ("Ursprung"), "Draw Area Size"=w111) -> (error out=w95:errorcluster)  [unwired: 2 in, 1 out]
      n104 = vi-ref "VisBx Anzeige.vi"() -> (w113:refnum<vi>)
      n105 = call "XML-String und Datei vergleichen.vi"("XML-String"=w109, "Datentypen aus Datei"=w108, "Namen aus Datei"=w104) -> ("nicht gleich"=w101:bool)  [unwired: 8 out]
      n106 = call "in Ursprung setzen.vi"("VI Referenz"=w113) -> ()  [unwired: 10 in, 1 out]
      n107 = property on="Fehler" class="Str"("Visible"=w101) -> (error out=w96:errorcluster)  [unwired: 2 in, 1 out]
      n108 = call "String in Array suchen.vi"("Nach String/Zeichen suchen (-)"="H2O", "String-Array"=w65) -> ("Index"=w69:i32)  [unwired: 7 in, 2 out]
      n109 = call "String in Array suchen.vi"("Nach String/Zeichen suchen (-)"="O2_25", "String-Array"=w65) -> ("Index"=w68:i32)  [unwired: 7 in, 2 out]
      n110 = call "String in Array suchen.vi"("Nach String/Zeichen suchen (-)"="THC_", "String-Array"=w65) -> ("Index"=w67:i32)  [unwired: 7 in, 2 out]
      n111 = Merge Errors(w27, w43, w42, w41, w93, w94, w85, w77, w76, w75) -> (w98:errorcluster)
      n112 = Merge Errors(w96, w95) -> (w97:errorcluster)
      n113 = call <vilib>:"Clear Errors.vi"("error in (no error)"=w97) -> ()  [unwired: 5 in, 2 out]
      n114 = Build Array(w69, w68, w67) -> (w66:i32[])
      n115 = call <vilib>:"Clear Errors.vi"("error in (no error)"=w98) -> ()  [unwired: 5 in, 2 out]
    }
  }
  n116 = while {
    tunnel: w2 -> [w165]
    tunnel: w1 -> [w162]
    stop <- FALSE stop-if-true
    n117 = event shown="[0] Timeout" {
      selector: _ -> [_ _ _ _]
      dyn-events: _ -> [_ _ _ _]
      timeout: 400 -> [_ _ _ _]
      tunnel: w165 -> [w217 _ _ _]
      tunnel: w162 -> [w188 _ _ _]
      event Timeout {
        # "aktuelle Werte für\nProzessvariable\naus XML-Daten"
        # "Bewegtbild bei jeder\nÄnderung neu zeichnen"
        n118 = event-data() -> ()  [unwired: 1 in, 3 out]
        n119 = call "FGV Messdaten.vi"("Aktionen"=Aktionen_FGV_Messdaten."lesen") -> ("Messdaten"=w182:sgl[][])  [unwired: 6 in, 8 out]
        n120 = disable-structure shown="Deaktiviert" {
          frame Disabled {
          }
          frame Enabled {
            n121 = disable-structure shown="Aktiviert" {
              disable-tunnel: [w228 TRUE] -> w224
              disable-tunnel: [w227 TRUE ("Amium AK Komm")] -> w223
              disable-tunnel: [w226 TRUE] -> w222
              frame Enabled {
                n122 = call "FGV System.vi"("Aktionen"=Aktioen_FGV_System."lesen") -> ("Optionen"=w229:T15)  [unwired: 12 in, 6 out]
                n123 = Unbundle By Name(w229) -> ("PNS?"=w225:bool)
                n124 = case shown="True" w225 {
                  selector: w225 -> [w232 w239]
                  tunnel: [w232 w234] -> w226
                  tunnel: [FALSE w235] -> w227
                  tunnel: [w231 w238] -> w228
                  frame False {
                    n125 = Not(x=w232) -> (.not. x?=w231:bool)
                  }
                  frame True {
                    n126 = call "Kommunikation Stoerung.vi"("Aktionen"=Aktionen_Kommunikation_Stoerung."lesen") -> ("Störung Messgerät"=w236:T26)  [unwired: 10 in]
                    n127 = Unbundle By Name(w236) -> ("Amium AK Komm"=w235:bool)
                    n128 = Not(x=w239) -> (.not. x?=w238:bool)
                    n129 = Not(x=w235) -> (.not. x?=w234:bool)
                  }
                }
              }
              frame Disabled {
              }
            }
            n130 = property on="VFS - FEHLER" class="Bool. (strikt)"("Visible"=w223) -> (error out=w220:errorcluster)  [unwired: 2 in, 1 out]
            n131 = property on="VFS - Aktiv" class="Bool. (strikt)"("Visible"=w222) -> (error out=w219:errorcluster)  [unwired: 2 in, 1 out]
            n132 = property on="VFS - Inaktiv" class="Bool. (strikt)"("Visible"=w224) -> (error out=w221:errorcluster)  [unwired: 2 in, 1 out]
            n133 = Merge Errors(w219, w220, w221) -> (w218:errorcluster)
            n134 = call <vilib>:"Clear Errors.vi"("error in (no error)"=w218) -> ()  [unwired: 5 in, 2 out]
          }
        }
        n135 = call "Vorschau Stoermeldungen.vi"() -> ("Vorschau Störungen"=→"Aktive Störungen":string[])  [unwired: 10 in, 1 out]
        n136 = call "FGV PNS Istwerte.vi"("Aktionen"=Aktionen_FGV_Istwerte."lesen") -> ("Regler"=w171:T27)  [unwired: 11 in, 3 out]
        n137 = call "VI Anlagenuebersicht.vi"() -> ("XML-String"=w206:string)  [unwired: 11 in]
        n138 = call "FGV cRIO-Daten.vi"("Aktion"=enum16{"lesen", "schreiben"}."lesen") -> ("Analog Input"=w210:T28, "TC Eingänge"=w191:T29)  [unwired: 9 in, 8 out]
        n139 = call "FGV Amium Daten.vi"("Aktion"=Aktion_FGV_Amium_Daten."lesen") -> ("Amium Daten"=w180:T30)  [unwired: 9 in, 5 out]
        n140 = call "XML-String in Werte-Array.vi"("XML-String"=w206) -> ("Werte"=w207:string[])
        n141 = call "FGV cRIO-Daten.vi"("Aktion"=enum16{"lesen", "schreiben"}."lesen") -> ("Betriebsstunden"=w199:sgl[])  [unwired: 9 in, 9 out]
        n142 = Index Array(array=w171) -> (element #1=w172:T32, element #2=w173:T32, element #3=w174:T32, element #4=w175:T32)  [unwired: 4 in]
        n143 = for {
          tunnel: [w246] -> w186 mode=indexing
          tunnel: w188 -> [w243] mode=indexing
          tunnel: w182 -> [w244]
          n144 = Index Array(array=w244, index (col)=w243) -> (element=w245:sgl[])  [unwired: 1 in]
          n145 = Array Size(array=w245) -> (size(s)=w249:i32)
          n146 = Subtract(x=w249, y=1) -> (x-y=w247:i32)
          n147 = Index Array(array=w245, index=w247) -> (element=w246:sgl)
        }
        n148 = Unbundle By Name(w180) -> ("Messgasdruck"=→"kPa":sgl)
        n149 = Unbundle By Name(w210) -> ("AI0: Durchfluss FT-IR"=→"Durchfluss FT-IR:":sgl, "AI1: Druck Ausgang"=→"Druck Ausgang:":sgl, "AI4: Druck CalGas"=→"Druck CalGas:":sgl, "AI2: Umgebungsdruck"=→"Umgebungsdruck:":sgl)
        n150 = call "FGV cRIO-Daten.vi"("Aktion"=enum16{"lesen", "schreiben"}."lesen") -> ("DO 0-31"=w202:T33)  [unwired: 9 in, 9 out]
        n151 = Unbundle By Name(w191) -> ("TC10: Schaltschrank"=→"Schaltschrank:":sgl, "TC0: Reserve"=→"Filter:":sgl, "TC11: Umgebung"=→"Umgebungstemperatur:":sgl, "TC1: HL zu FT-IR"=→"HL zu FT-IR:":sgl, "TC2: HL Extern SP1"=→"HL Ext. SP1:":sgl, "TC3: HL Extern SP2"=→"HL Ext. SP2:":sgl)  [unwired: 1 out]
        n152 = Unbundle By Name(w202) -> ("O4: CG 4 (FB CalGas)"=w196:bool)
        n153 = for {
          shift-right: [w255] -> w205
          shift-left: w217 -> [w252]
          tunnel: w207 -> [w251] mode=indexing
          i -> [w250]
          # "Zeichenbefehle für jede\nProzessvariable i ermitteln"
          n154 = call "FGV Zuordnungstabelle Vis.vi"("Prozessvariable Nr. N"=w250, "Wert (N)"=w251) -> ("Wert für zeichnen"=w253:string, "Zeichenbefehle"=w254:T16[])  [unwired: 4 in, 4 out]
          n155 = for {
            tunnel: w253 -> [w256]
            tunnel: w254 -> [w257] mode=indexing
            shift-right: [w259] -> w255
            shift-left: w252 -> [w258]
            n156 = call "Vis-Element zeichnen.vi"("Wert-String"=w256, "Schritt"=w257, "Bild alt"=w258) -> ("Bild neu"=w259:picture)  [unwired: 4 in, 4 out]
          }
        }
        "Bild" <- w205
        n157 = Unbundle By Name(w172) -> ("Istwert"=→"Filterblock PNS":i16)
        n158 = Unbundle By Name(w173) -> ("Istwert"=→"Heizleitung SP1:":i16)
        n159 = Unbundle By Name(w174) -> ("Istwert"=→"Heizleitung SP2:":i16)
        n160 = Unbundle By Name(w175) -> ()  [unwired: 1 out]
        n161 = Index Array(array=w199) -> (element #1=→"Betriebsstunden Pumpe:":sgl, element #2=→"Betriebsstunden Anlage:":sgl)  [unwired: 2 in]
        n162 = call "FGV FT-IR Diagnosewerte.vi"("Aktionen"=FGV_FT-IR_Diagnose_Aktionen."Lesen") -> ("Druck"=→"Eingangsdruck FT-IR:":dbl, "Temperatur"=→"Temp. Messzelle:":dbl)  [unwired: 5 in, 4 out]
        n163 = Select(t=T9."Enabled", s=w196, f=T9."Disabled and Grayed Out" ("Deaktiviert")) -> (s? t:f=w195:T9)
        n164 = property on="Druck CalGas:" class="DigWert (strikt)"("DisabledEnum"=w195) -> (error out=w194:errorcluster)  [unwired: 2 in, 1 out]
        n165 = Index Array(array=w186) -> (element #1=→"H2O":sgl, element #2=→"O2":sgl, element #3=→"HC":sgl)  [unwired: 3 in]
        n166 = call "Uebersicht Ausgabefelder einfaerben.vi"("Aktionen"=Aktionen_Ausgabefaelder_einfaerben."prüfen") -> ()  [unwired: 11 in]
        n167 = call <vilib>:"Clear Errors.vi"("error in (no error)"=w194) -> ()  [unwired: 5 in, 2 out]
      }
      event "CG-Test": Value Change {
        n168 = event-data() -> ()  [unwired: 1 in, 6 out]
        n169 = vi-ref "Erweiterte Konfig.lvlib:CG-Check Konfig.lvlib:CG-Test.vi"() -> (w260:refnum<vi>)
        n170 = call "VI Pop Up.vi"("VI Referenz"=w260) -> ()  [unwired: 10 in, 1 out]
      }
      event "N2 zu PNS": Value Change {
        n171 = event-data() -> ()  [unwired: 1 in, 1 out]
        n172 = call "FGV-Erweiterte Bedienung.vi"("Aktion"=FGV_Erweiterte_Bedienung_Aktion."Lesen") -> ("N2 zu PNS"=w262:bool)  [unwired: 9 in, 1 out]
        n173 = Not(x=w262) -> (.not. x?=w261:bool)
        n174 = call "FGV-Erweiterte Bedienung.vi"("Aktion"=FGV_Erweiterte_Bedienung_Aktion."N2 zu PNS", "N2 zu PNS"=w261) -> ()  [unwired: 8 in, 2 out]
      }
      event "VFS": Value Change {
        n175 = event-data() -> ()  [unwired: 1 in, 1 out]
        n176 = disable-structure shown="Amium_PNS_aktiv==FALSE, Standard" {
          disable-tunnel: [w266 w267] -> w265
          frame condition #0 {
            n177 = vi-ref "Amium PNS.lvlib:Anlagenuebersicht_amium2.vi"() -> (w266:refnum<vi>)
          }
          frame condition #1 (active) {
            n178 = vi-ref "PNS.lvlib:PNS Anlagenuebersicht.lvlib:VisBx Anzeige PNS.vi"() -> (w267:refnum<vi>)
          }
        }
        n179 = call "VI Pop Up.vi"("VI Referenz"=w265) -> ()  [unwired: 10 in, 1 out]
      }
    }
  }
  n180 = disable-structure shown="Deaktiviert" {
    frame Disabled {
      n181 = flat-sequence {
        frame #0 {
          w268 = TRUE ("Sichtbar")
          n182 = property on="HL Ext.:" class="DigWert (strikt)"("Visible"=w268) -> ()  [unwired: 2 in, 2 out]
          n183 = property on="Druck CalGas:" class="DigWert (strikt)"("Visible"=w268) -> ()  [unwired: 2 in, 2 out]
        }
      }
    }
    frame Enabled {
    }
  }
